vi "Untitled 43.vi"(8 "error in":errorcluster) -> (0 "error out":errorcluster, 3 "task out":refnum<k21>)   [LabVIEW 2019]
uses:
  <vilib>/DAQmx/create/channels.llb/DAQmx Create Channel (AO-Voltage-Basic).vi
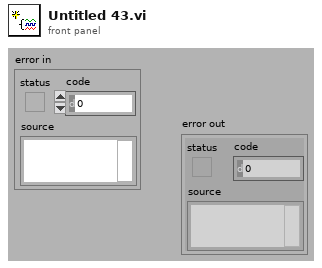
[diagram p1: front panel]
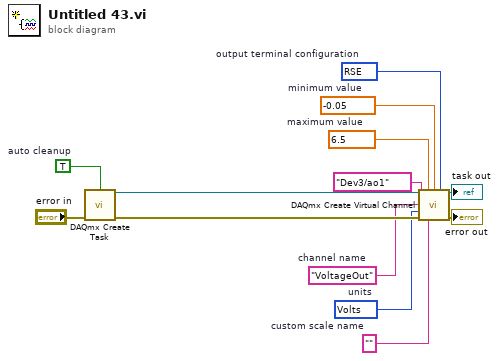
[diagram p0: block diagram]
diagram:
  w2 = 10083 items=["Default"=-1, "RSE"=10083, "Differential"=10106, "Pseudodifferential"=12529]  # output terminal configuration
  w3 = 10348 items=["Volts"=10348, "From Custom Scale"=10065]  # units
  w4 = "VoltageOut"  # channel name
  w7 = ""  # custom scale name
  w8 = -0.05  # minimum value
  w9 = 6.5  # maximum value
  w11 = TRUE  # auto cleanup
  n1 = call <vilib>:"DAQmx Create Task.vi"("auto cleanup"=w11, "error in"="error in") -> ("task out"=w10:refnum<k21>, "error out"=w12:errorcluster)  [unwired: 12 in]
  n2 = call-poly <vilib>:"DAQmx Create Virtual Channel.vi"("task in"=w10, "maximum value"=w9, "minimum value"=w8, "output terminal configuration"=w2, "physical channels"=tag "Dev3/ao1", "name to assign"=w4, "units"=w3, "error in"=w12, "custom scale name"=w7) -> ("task out"=→"task out":refnum<k21>, "error out"=→"error out":errorcluster)  [unwired: 5 in]
